vi "Engine-Channels-Host.vi"() -> ()   [LabVIEW 2016]
uses:
  Shared/Typedefs/Engine-Channel-Array.ctl
  Shared/Typedefs/Engine-Channel.ctl
  Shared/DSI-Shared.lvlib
panel:
  out "ENG|Channels|Data":T1
  in  "_DSI Channel Data":i32(listbox) caption="DSI Channel Data"
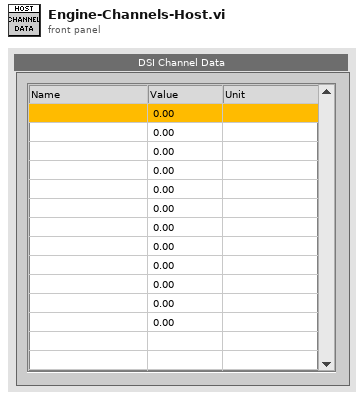
[diagram p1: front panel]
types:
  T1 = typedef "DSI-Shared.lvlib/Engine-Channel-Array.ctl" = T2[]
  T2 = typedef "DSI-Shared.lvlib/Engine-Channel.ctl" = cluster{"Name":string, "Unit":string, "Value":sgl}
  T3 = typedef "LVRectTypeDef.ctl" = cluster{"Left":i16, "Top":i16, "Right":i16, "Bottom":i16}
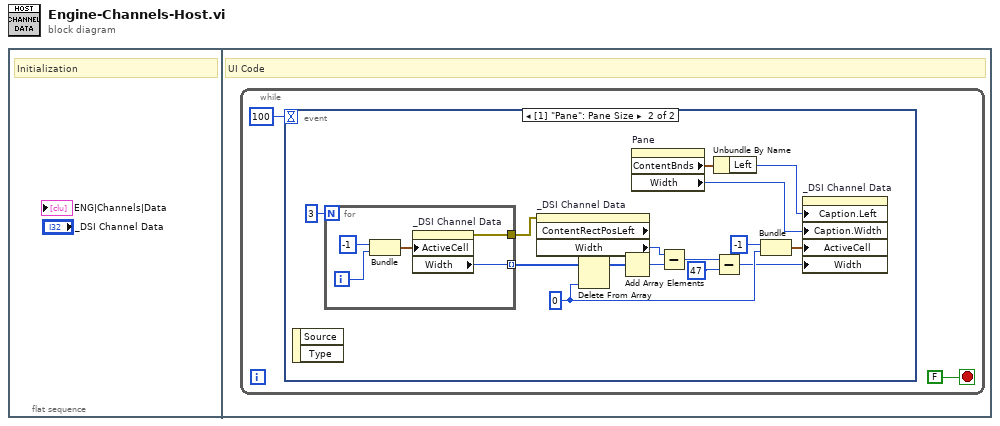
[diagram p0: block diagram]
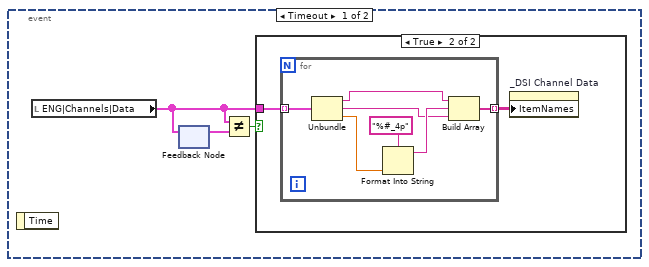
[diagram p2: hidden frame]
diagram:
  n1 = flat-sequence {
    frame #0 {
      # "Initialization"
    }
    frame #1 {
      # "UI Code"
      n2 = while {
        stop <- FALSE stop-if-true
        n3 = event shown="[1] \"Pane\": Pane Size" {
          selector: _ -> [_ _]
          dyn-events: _ -> [_ _]
          timeout: 100 -> [_ _]
          event Timeout {
            n4 = event-data() -> ()  [unwired: 1 in, 1 out]
            n5 = local read "ENG|Channels|Data"() -> (w3:T1)
            n6 = feedback-in #1(w3) -> ()
            n7 = feedback #1() -> (w4:T1)  [unwired: 1 in]
            n8 = Not Equal?(x=w3, y=w4) -> (x != y?=w5:bool)
            n9 = case shown="True" w5 {
              tunnel: w3 -> [_ w7]
              frame False {
              }
              frame True {
                n10 = for {
                  tunnel: w7 -> [w14] mode=indexing
                  tunnel: [w10] -> w6 mode=indexing
                  n11 = Unbundle(w14) -> ("Name"=w11:string, "Unit"=w8:string, "Value"=w12:sgl)
                  n12 = Format Into String(format string="%#_4p", w12) -> (resulting string=w9:string)  [unwired: 2 in, 1 out]
                  n13 = Build Array(w11, w9, w8) -> (w10:string[])
                }
                n14 = property on="_DSI Channel Data" class="MCListbox (strict)"("ItemNames"=w6) -> ()  [unwired: 2 in, 2 out]
              }
            }
          }
          event Pane Size {
            w23 = 0 ("index")
            n15 = event-data() -> ()  [unwired: 1 in, 2 out]
            n16 = for {
              N: 3 -> [_]
              tunnel: [w31] -> w28 mode=indexing
              tunnel: [w30] -> w29
              i -> [w33]
              n17 = Bundle(-1, w33) -> (w34:cluster{i32, i32})  [unwired: 1 in]
              n18 = property on="_DSI Channel Data" class="MCListbox (strict)"("ActiveCell"=w34) -> (error out=w30:errorcluster, "Width"=w31:u32)  [unwired: 2 in, 1 out]
            }
            n19 = property on="_DSI Channel Data" class="MCListbox (strict)" props=["ContentRectPosLeft", "Width"](error in=w29) -> ("Width"=w18:u32)  [unwired: 1 in, 3 out]
            n20 = Delete From Array(array=w28, index=w23) -> (array with subset deleted=w27:u32[])  [unwired: 1 in, 1 out]
            n21 = Add Array Elements(numeric array=w27) -> (sum=w26:u32)
            n22 = property on="Pane" class="Pane"() -> ("ContentBnds"=w16:T3, "Width"=w17:u32)  [unwired: 2 in, 2 out]
            n23 = Subtract(x=w18, y=w26) -> (x-y=w25:u32)
            n24 = Unbundle By Name(w16) -> ("Left"=w15:i16)
            n25 = Subtract(x=w25, y=u32 47) -> (x-y=w21:u32)
            n26 = Bundle(-1, "index"=w23) -> (w22:cluster{i32, "index":i32})  [unwired: 1 in]
            n27 = property on="_DSI Channel Data" class="MCListbox (strict)"("Caption.Left"=w15, "Caption.Width"=w17, "ActiveCell"=w22, "Width"=w21) -> ()  [unwired: 2 in, 2 out]
          }
        }
      }
    }
  }
